vi "checkFinishEnemyPossessionAtOurField.vi"(8 "error in (no error)":errorcluster, 9 "last command_interpreted":T1, 10 "Game":refnum<class "Game.lvclass">, 11 "EnemyPossessionAtOurFieldPlay in":refnum<class "EnemyPossessionAtOurFieldPlay.lvclass">) -> (0 "error out":errorcluster, 2 "finish":bool, 3 "EnemyPossessionAtOurFieldPlay out":refnum<class "EnemyPossessionAtOurFieldPlay.lvclass">)   [LabVIEW 2024, in "EnemyPossessionAtOurFieldPlay.lvclass"]
uses:
  EnemyPossessionAtOurFieldPlay.lvclass
  Game_class/Game.lvclass
  Referee_class/command_interpreted.ctl
  Events_class/Possession.ctl
  Game_class/Game.lvclass/Game.ctl
  Referee_class/Referee.lvclass/Referee.ctl
  Ball_class/Ball.lvclass/Ball.ctl
  Events_class/Events.lvclass/Events.ctl
  Game_class/Read Referee.vi
  Game_class/Read EventsRef.vi
  Game_class/Read BallRef.vi
  Game_class/Read Utilities.lvclass.vi
  Game_class/Read AllyRef.vi
  Game_class/Read EnemyRef.vi
  Game_class/Read NewParameters.vi
  Ball_class/Read v_x.vi
  Ball_class/Read v_y.vi
  Events_class/Read ball_out.vi
  Events_class/Read touch.vi
  Events_class/Read id_touch.vi
  Referee_class/Read command_interpreted.vi
  Referee_class/Referee.lvclass
  Events_class/Events.lvclass
  Ball_class/Ball.lvclass
  Utilities_class/Utilities.lvclass
  Ally_class/Ally.lvclass
  Enemy_class/Enemy.lvclass
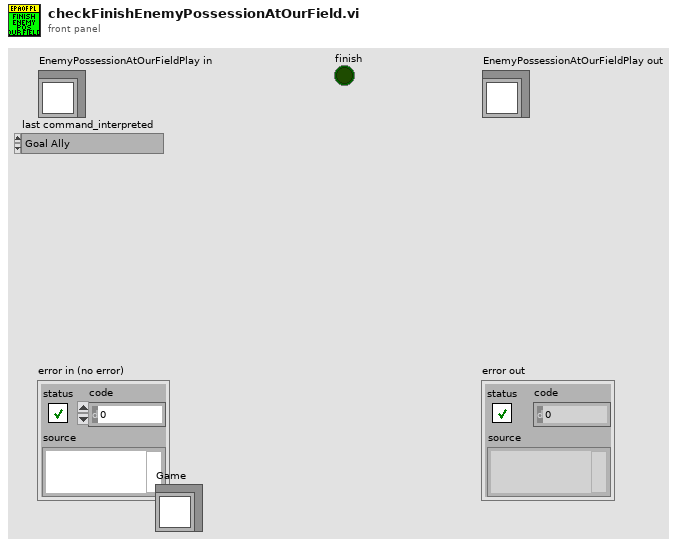
[diagram p1: front panel]
types:
  T1 = typedef "command_interpreted.ctl" = enum16{"Goal Ally", "Goal Enemy", "Ball Placement Enemy", "Ball Placement Ally", "Normal Half Time", "Extra Time  Break", "Extra Half Time", "None", "Post Game", "PKA Normal Start", "Prepare Kickoff Ally", "PKE Normal Start", "Prepare Kickoff Enemy", "Force Start", "Halt", "Timeout", "Prepare Penalty Ally", "Prepare Penalty Enemy", "PPA NormalStart", "PPE Normal Start", "Indirect Free Ally", "Direct Free Enemy", "Direct Free Ally", "Indirect Free Enemy", "Stop"}
  T2 = typedef "Events.lvclass/Possession.ctl" = enum16{"OurPossession", "TheirPossession", "Contended", "Loose"}
  T3 = typedef "NewParameters.ctl" = cluster{"PenaltyDistance":dbl, "DistanceAttackerToBackBall":dbl, "Division":enum16{"Div B", "Div A"}, "DistanceToAvoidyEnemyRobot":dbl, "BallPlacementDistance":dbl, "DisatanceBehindBallToStealBall":dbl, "MaxDistanceToPositionKickoff":dbl, "BlockEnemyTarget":bool, "MaxStopVAng":dbl, "DistanceMarkerToEnemy":dbl, "IgnoreDribblerContact":bool, "DistanceToBeginEnemyPosession":dbl, "GoToBallWhenEnemyNotMoving":bool, "EnemyDistanceToReduceVelocity":dbl, "TurnOnEnemyDistanceToReduceVelocity":bool, "EnemyDistanceToShootOutBall":dbl, "DefenseKickBall":bool, "MoreKickToGoal? (0-0.3)":dbl, "ChipKickInEnemyField":bool, "ShootOutRobotId":dbl, "FieldLenghtDenominatorInShootOut":dbl, "AdjustPositionInBallPlacement":bool, "PowerGodPass":dbl, "VelocityAbortEnemyPos":dbl, "MaxDistToBeginPass":dbl, "MinDistToBeginPass":dbl, "VelocityInDirects":dbl, "BadDribblerIDs":i32[], "NewKickToDistanceAroundBall":dbl, "PowerAvoidColisionMarker":dbl, "DistanceToAvoidColisionMarker":dbl, "AvoidBallKick":dbl, "DistanceTryKick":dbl, "SuicideKickDIstance":dbl, "AdjustFirstKickDistance":dbl, "AvoidAimLessKick":dbl, "DistanceToAvoidyEnemyShootRobot ":dbl, "NumberOfMarkers":dbl, "PotField":bool, "PIDLateral":bool, "MinDistanceFirstKickX":dbl, "MinDistanceFirstKickY":dbl, "FractionOfDistToTouchGround\nAfterChipKick":dbl, "FractionOfKickxWhen\nComposedWithKickz":dbl, "Style":T4, "MoveInTurnState":bool, "DistFromEnemyToConsider\nMoveInTurnState":dbl, "CascadePID":bool, "TurnAroundParameters":cluster{"Radius":dbl, "Multiplier":dbl, "ChordAngle":dbl}, "SafeDriveVel":dbl, "DistanceToGoToBackBall":dbl, "minDistanceToNotFinish\nEnemyPossession":dbl, "OneTouchShot":cluster{"angleFactor":dbl, "maxAngle":dbl, "Attack":bool, "Defense":bool}, "OpenAngleToGoal":cluster{"minAngle":dbl, "maxAngle":dbl, "minEvaluation":dbl}, "ShotInterception":cluster{"shotSpeed":dbl, "minEnemySpeed":dbl, "maxEnemySpeed":dbl, "minEvaluation":dbl}, "AllyTeamArray":T5[], "maxDefendersNumber":i32, "Zone":cluster{"GuardPositionArray":dbl[][], "ZoneMidField":dbl[], "CenterForwardWidth":dbl}, "MinEvaluationToShoot":dbl, "PassInterception":cluster{"maxPassSpeed":dbl, "minPassSpeed":dbl, "minEnemySpeed":dbl, "chipPassDistance":dbl, "chipPassEvaluation":dbl, "minEvaluation":dbl, "maxEnemySpeed":dbl}, "PassDistance":cluster{"maxDistance":dbl, "minDistance":dbl}, "receiverSpeed":dbl, "maxBallSpeed":dbl, "slackTime":dbl, "Turning radius":dbl, "Turning v_ang":dbl, "AlignError":cluster{"Distance":dbl, "Orientation":dbl, "V_norm(m/s)":dbl, "V_ang (rad/s)":dbl}, "RobotRadius":dbl, "KickerDistance":dbl, "keeper angle  to cover goalpost":dbl, "a_slide":dbl, "a_roll":dbl, "k_switch":dbl}
  T4 = typedef "Style.ctl" = enum16{"Insanity", "Offensive", "Defensive"}
  T5 = typedef "AllyTeam.ctl" = enum16{"Keeper", "Defender", "Attacker"}
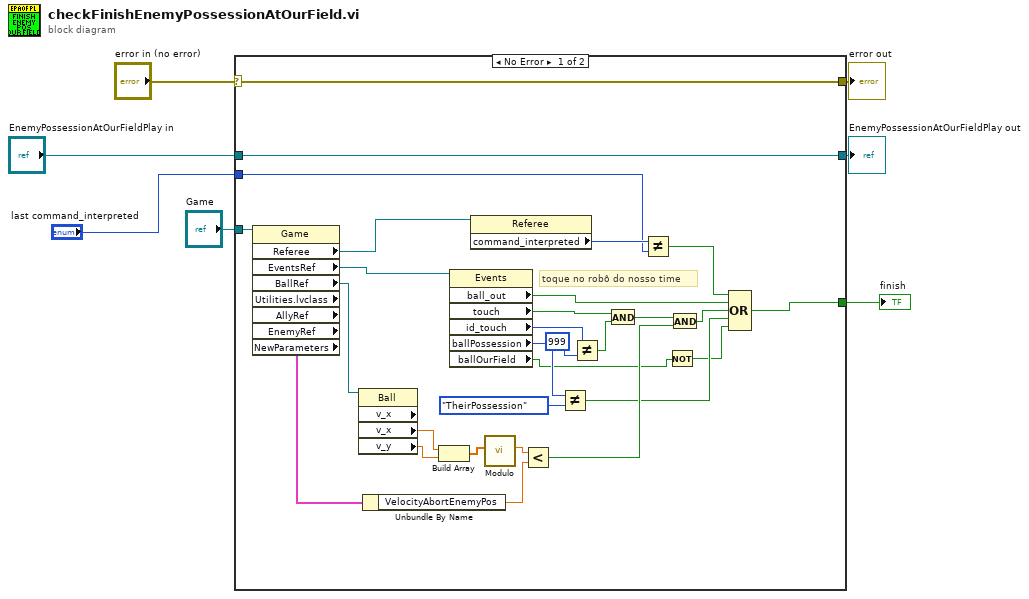
[diagram p0: block diagram]
diagram:
  n1 = case shown="No Error" "error in (no error)" {
    selector: "error in (no error)" -> [w35 w38]
    tunnel: [w35 w38] -> w6
    tunnel: [w36 w37] -> w4
    tunnel: "EnemyPossessionAtOurFieldPlay in" -> [w36 w37]
    tunnel: "Game" -> [w29 _]
    tunnel: [w16 _] -> w2
    tunnel: "last command_interpreted" -> [w28 _]
    frame No Error {
      # "toque no robô do nosso time"
      n2 = property class="Game" props=["Referee", "EventsRef", "BallRef", "Utilities.lvclass", "AllyRef", "EnemyRef", "NewParameters"](reference=w29) -> ("Referee"=w34:refnum<class "Referee.lvclass">, "EventsRef"=w32:refnum<class "Events.lvclass">, "BallRef"=w24:refnum<class "Ball.lvclass">, "NewParameters"=w21:T3)  [unwired: 1 in, 5 out]
      n3 = property class="Ball" props=["v_x", "v_x", "v_y"](reference=w24) -> ("v_x"=w18:dbl, "v_y"=w17:dbl)  [unwired: 1 in, 3 out]
      n4 = Unbundle By Name(w21) -> ("VelocityAbortEnemyPos"=w20:dbl)
      n5 = Build Array(w18, w17) -> (w23:dbl[])
      n6 = property class="Events"(reference=w32) -> ("ball_out"=w30:bool, "touch"=w27:bool, "id_touch"=w19:i32, "ballPossession"=w12:T2, "ballOurField"=w9:bool)  [unwired: 1 in, 2 out]
      n7 = property class="Referee"(reference=w34) -> ("command_interpreted"=w33:T1)  [unwired: 1 in, 2 out]
      n8 = call "Modulo.vi"("2D vector"=w23) -> ("Modulo"=w22:dbl)  [unwired: 10 in]
      n9 = Less?(x=w22, y=w20) -> (x < y?=w13:bool)
      n10 = Not Equal?(x=w12, y=Possession."TheirPossession") -> (x != y?=w10:bool)
      n11 = Not Equal?(x=w19, y=999) -> (x != y?=w26:bool)
      n12 = And(x=w27, y=w26) -> (x .and. y?=w15:bool)
      n13 = Not Equal?(x=w33, y=w28) -> (x != y?=w31:bool)
      n14 = Not(x=w9) -> (.not. x?=w8:bool)
      n15 = And(x=w15, y=w13) -> (x .and. y?=w14:bool)
      n16 = Compound Arithmetic op=OR(w31, w30, w14, w10, w8) -> (w16:bool)
    }
    frame Error {
    }
  }
  "error out" <- w6
  "EnemyPossessionAtOurFieldPlay out" <- w4
  "finish" <- w2
